vi "Modbus_Get_Time.vi"(8 "error in (no error)":errorcluster, 11 "TCP Network Connection in":refnum<k5>) -> (0 "error out":errorcluster, 1 "Time Stamp":timestamp, 2 "Slave Input Registers":u16[](array[numeric]) caption="Data Time Registers", 3 "TCP Network Connection out":refnum<k5>)   [LabVIEW 2014]
uses:
  <vilib>/NI Modbus.llb/MB Ethernet Master Query Read Holding Registers (poly).vi
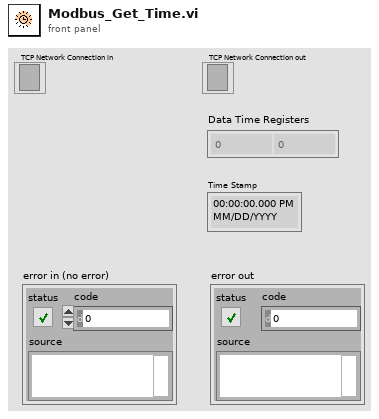
[diagram p1: front panel]
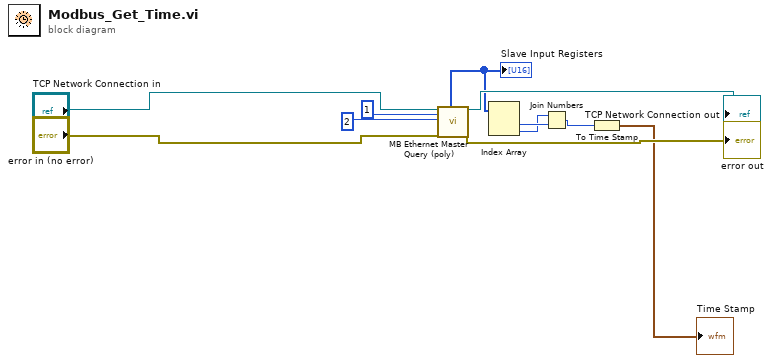
[diagram p0: block diagram]
diagram:
  n1 = call-poly <vilib>:"MB Ethernet Master Query (poly).vi"("TCP Connection Refnum in"="TCP Network Connection in", "Starting Address"=u16 1, "Quantity"=u16 2, "error in"="error in (no error)") -> ("TCP Connection Refnum (dup)"=→"TCP Network Connection out":refnum<k5>, "Holding Registers"=w5:u16[], "error out"=→"error out":errorcluster)  [unwired: 1 in, 12 out]
  "Slave Input Registers" <- w5
  n2 = Index Array(array=w5) -> (element #1=w9:u16, element #2=w8:u16)  [unwired: 2 in]
  n3 = Join Numbers(hi=w8, lo=w9) -> ((hi.lo)=w6:u32)
  n4 = To Time Stamp(1:w6) -> (0:→"Time Stamp":timestamp)
